vi "Main.vi"(11 "Module Admin":refnum<class "Delacor_lib_QMH_Module Admin.lvclass">) -> ()   [LabVIEW 2022 SP3, in "MainPanel.lvlib"]
doc: "This template is based off of the Queued Message Handler design pattern and the Queued Message Handler project template that ships with LabVIEW.\n\nThe main difference is that the queue is private to this module and communication between modules is performed via Broadcast and Request events.\n\nRequest events are wrapped in public API methods and are handled in the Event Handling Loop (EHL) of this VI. Any module can register for Broadcast events sent by this module. The EHL generates messages based on user interface actions.\n\nThe Message Handling Loop (MHL) processes messages generated by the EHL, or by other messages. The messages are string values, so new messages can be added easily to the Message Cases case structure in the MHL. Each message cluster can also provide an optional value for Message Data, which is a variant that can be converted to whatever message-specific data is required.\n_____\nBased on DQMH Project Template 7.0.1.1316."
uses:
  MainPanel.lvlib
  <vilib>/Delacor/Delacor QMH/Libraries/Module Admin_class/Delacor_lib_QMH_Module Admin.lvclass
  Module Data--cluster.ctl
  Do Something Argument--cluster.ctl
  <vilib>/Delacor/Delacor QMH/Libraries/Message Queue_class/Delacor_lib_QMH_Message Queue.lvclass/Delacor_lib_QMH_Message Queue.ctl
  Do Something Else Argument--cluster.ctl
  Do Something Else and Wait for Reply Argument--cluster.ctl
  Do Something Else and Wait (Reply Payload)--cluster.ctl
  Stop Argument--cluster.ctl
  <vilib>/Delacor/Delacor QMH/Libraries/Module Admin_class/Delacor_lib_QMH_Module Admin.lvclass/Delacor_lib_QMH_Module Admin.ctl
  Prepare Argument--cluster.ctl
  Configure Argument--cluster.ctl
  Request UI Display Argument--cluster.ctl
  Framework/UI Manager/Module Display Scenarios.ctl
  Request UI Display (Reply Payload)--cluster.ctl
  Update UI Argument--cluster.ctl
  <vilib>/Utility/miscctls.llb/LVPointTypeDef.ctl
  <vilib>/Delacor/Delacor QMH/Libraries/Message Queue_class/Delacor_lib_QMH_Enqueue Message (Single).vi
  <vilib>/Delacor/Delacor QMH/Libraries/Module Admin_class/Delacor_lib_QMH_Get External Launch.vi
  <vilib>/Delacor/Delacor QMH/Libraries/Message Queue_class/Delacor_lib_QMH_Message Queue.lvclass
  Libraries/hse-libraries/Source/hse-configuration/config-ini/config-ini.lvclass
  Framework/UI Manager/UI Manager.lvlib
  <vilib>/Hampel Software Engineering/HSE Logger/hse-logger.lvlib
  Libraries/hse-libraries/Source/hse-dqmh/hse-dqmh.lvlib
panel:
  in  "Run Model":bool
  out "error out":errorcluster
  out "X":dbl
  out "Status":string
  in  "Simulate MHL Error":bool
  in  "Simulate EHL Error":bool
  in  "Do Something Else <Replace Me>":bool
  in  "Do Something <Replace Me>":bool
  # "These controls have associated \"Value Changed\" events configured in the Event Structure on the diagram.\n\nReplace them (and reconfigure the Event Structure) with the controls you need for your application. \n\nOther processes communicate with this Module via its Public API (wrappers for its Request Events).\n\nThis Module communicates with other processes via its Broadcast Events.\nAny process that wants to receive these messages can register for this module's Broadcast events."
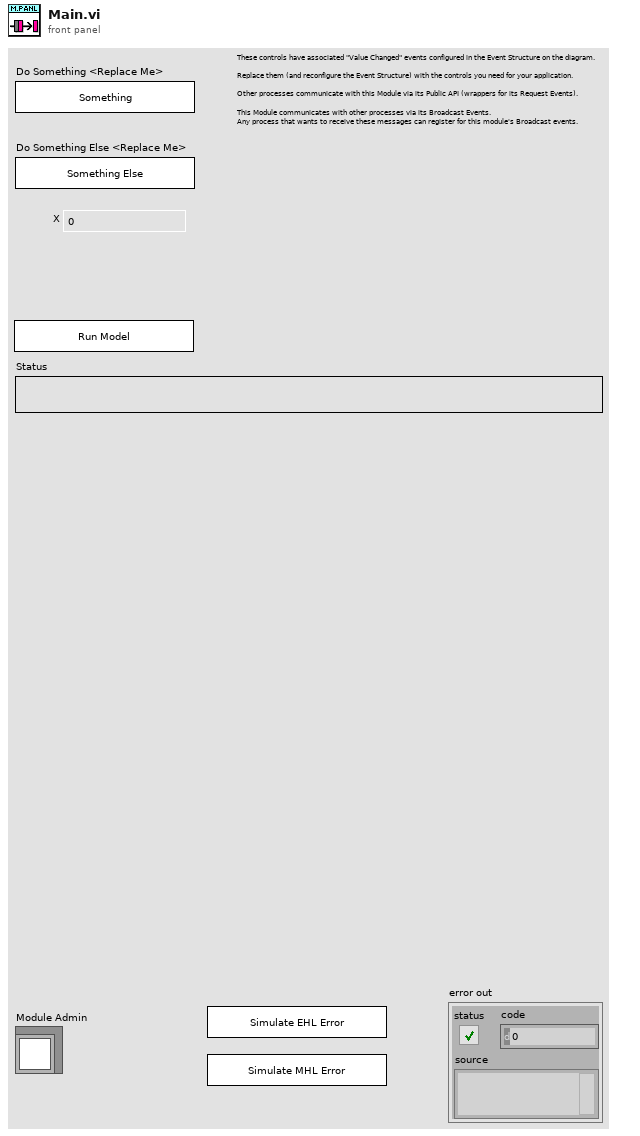
[diagram p1: front panel]
types:
  T1 = typedef "MainPanel.lvlib/Request Events--cluster.ctl" = cluster{"Stop Module":refnum<user-event>, "Do Something":refnum<user-event>, "Do Something Else":refnum<user-event>, "Do Something Else and Wait for Reply":refnum<user-event>, "Show Panel":refnum<user-event>, "Hide Panel":refnum<user-event>, "Get Module Execution Status":refnum<user-event>, "Show Diagram":refnum<user-event>, "Prepare":refnum<user-event>, "Configure":refnum<user-event>, "Request UI Display":refnum<user-event>, "Private":cluster{"Update UI":refnum<user-event>}}
  T2 = typedef "MainPanel.lvlib/Module Data--cluster.ctl" = cluster{"Status":string, "Py Session":refnum<k35>, "Py Script Path":path}
  T3 = typedef "MainPanel.lvlib/Do Something Argument--cluster.ctl" = cluster{"Do Something Msg":string}
  T4 = typedef "MainPanel.lvlib/Do Something Else Argument--cluster.ctl" = cluster{"Do Something Else Msg":string, "X":dbl}
  T5 = typedef "MainPanel.lvlib/Do Something Else and Wait for Reply Argument--cluster.ctl" = cluster{"Do Something Else Msg":string, "X":dbl, "Wait Notifier":refnum<notifier>, "wait for reply":bool}
  T6 = enum32{"invalid lock state", "Not Locked", "Locked (No Password)", "Password-protected"}
  T7 = typedef "MainPanel.lvlib/Stop Argument--cluster.ctl" = cluster{"Origin":string, "Exit via Stop Module Req?":bool, "Wait for Module to stop?":bool}
  T8 = typedef "MainPanel.lvlib/Prepare Argument--cluster.ctl" = cluster{"Boolean":bool}
  T9 = typedef "MainPanel.lvlib/Configure Argument--cluster.ctl" = cluster{"Boolean":bool}
  T10 = typedef "MainPanel.lvlib/Request UI Display Argument--cluster.ctl" = cluster{"Scenario":T11, "Wait Notifier":refnum<notifier>, "wait for reply":bool}
  T11 = typedef "UI Manager.lvlib/Module Display Scenarios.ctl" = enum16{"Stand-Alone", "Managed"}
  T12 = typedef "MainPanel.lvlib/Update UI Argument--cluster.ctl" = cluster{"Update":bool}
  T13 = typedef "LVPointTypeDef.ctl" = cluster{"Horizontal":i16, "Vertical":i16}
  T14 = enum32{"Invalid", "Standard", "Closed", "Hidden", "Minimized", "Maximized"}
  T15 = typedef "MainPanel.lvlib/Do Something Else and Wait (Reply Payload)--cluster.ctl" = cluster{"Value":dbl, "error":errorcluster}
  T16 = typedef "MainPanel.lvlib/Request UI Display (Reply Payload)--cluster.ctl" = cluster{"Accept":bool, "error":errorcluster}
  T17 = typedef "hse-dqmh.lvlib/System Message Source.ctl" = enum16{"module", "application", "network"}
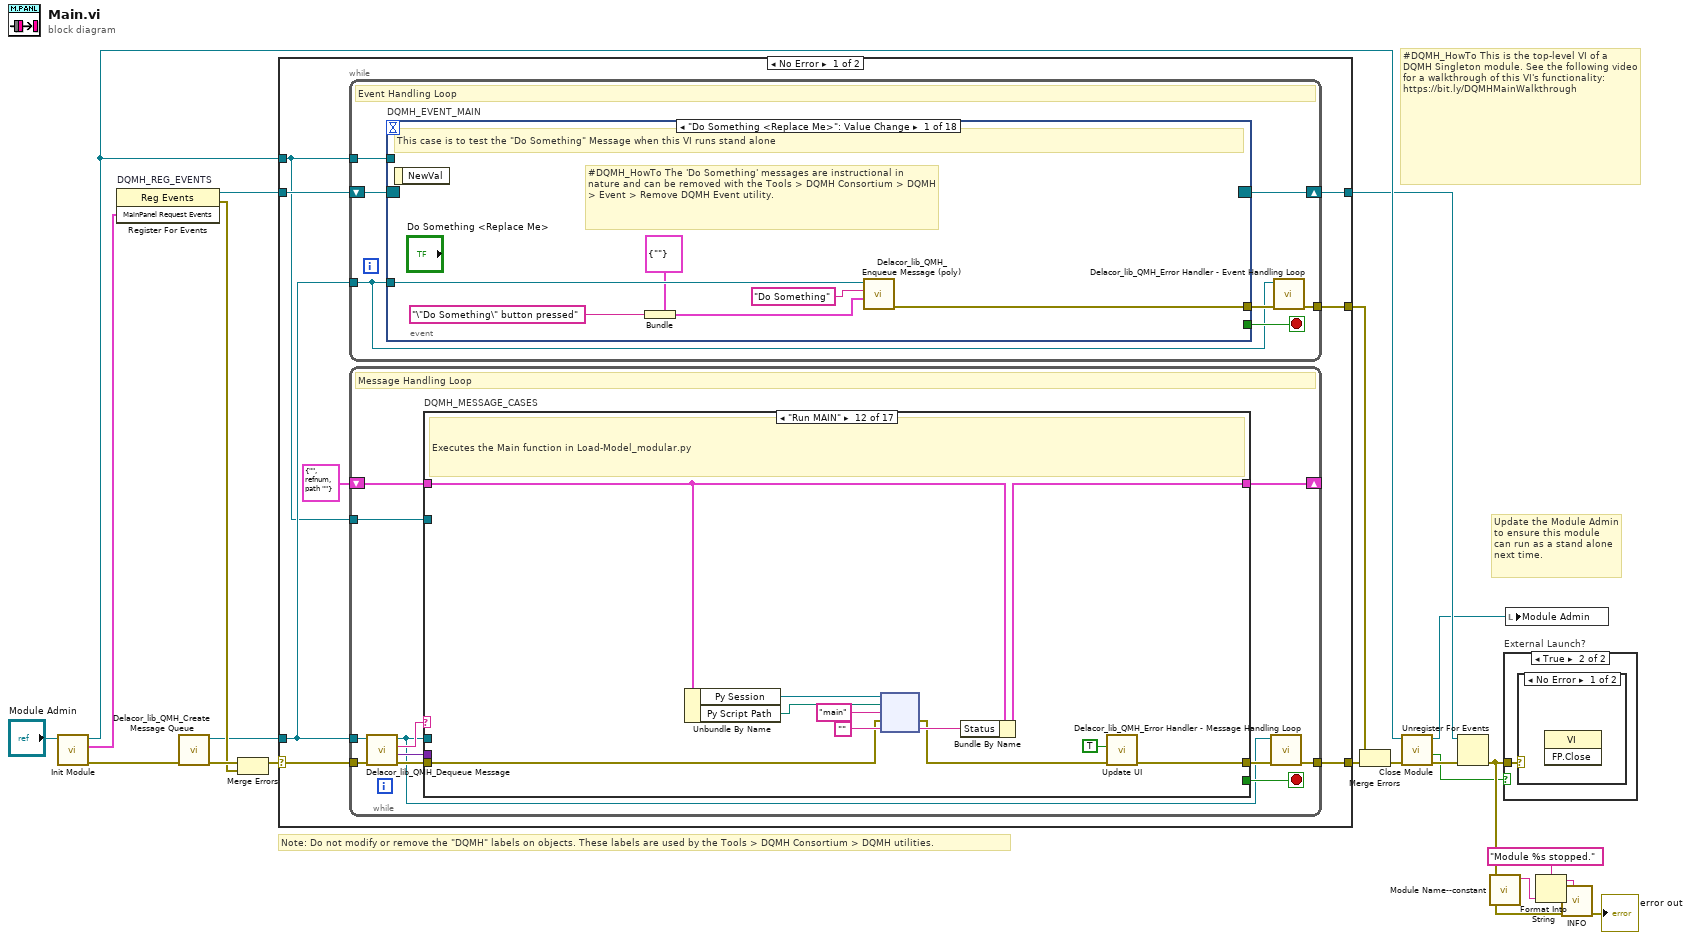
[diagram p0: block diagram]
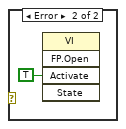
[diagram p3: hidden frame]
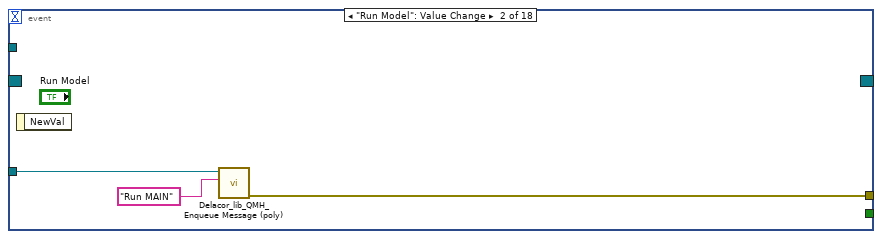
[diagram p4: hidden frame]
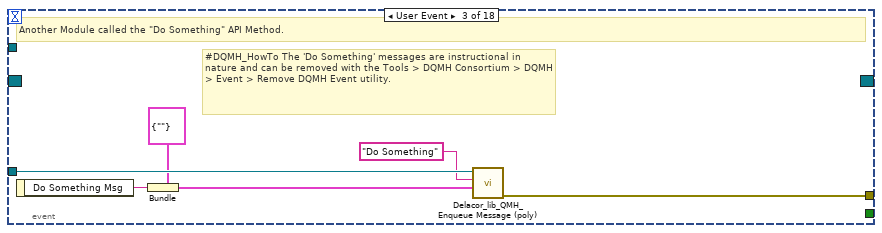
[diagram p5: hidden frame]
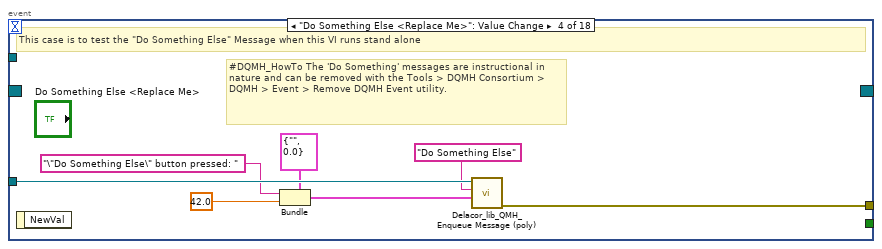
[diagram p6: hidden frame]
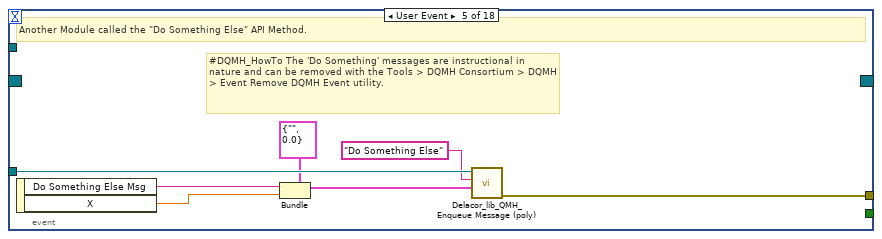
[diagram p7: hidden frame]
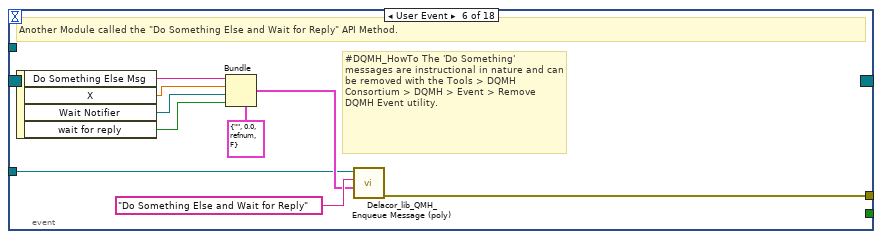
[diagram p8: hidden frame]
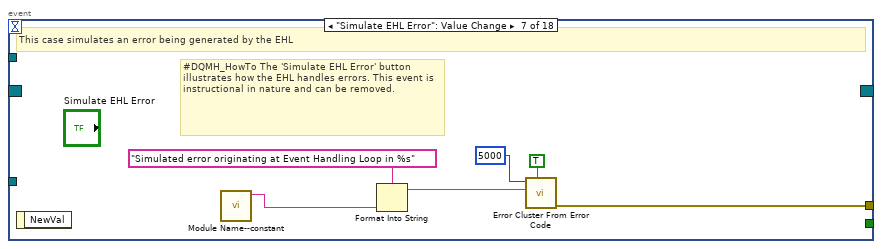
[diagram p9: hidden frame]
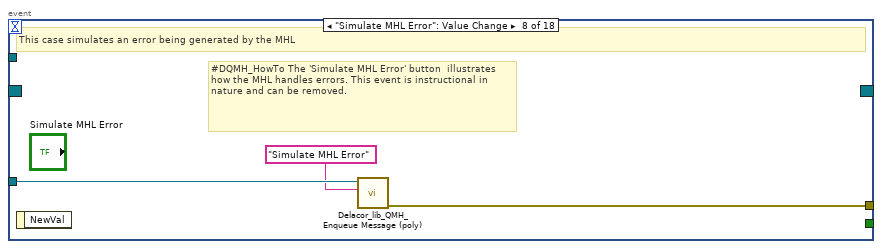
[diagram p10: hidden frame]
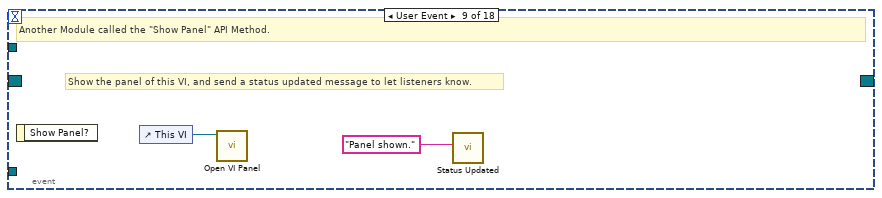
[diagram p11: hidden frame]
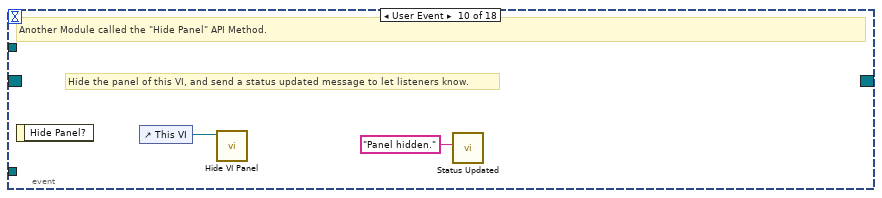
[diagram p12: hidden frame]
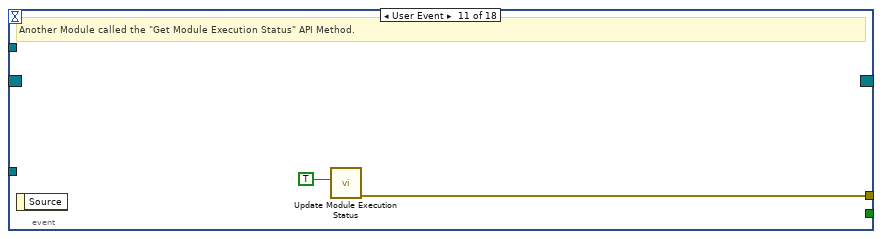
[diagram p13: hidden frame]
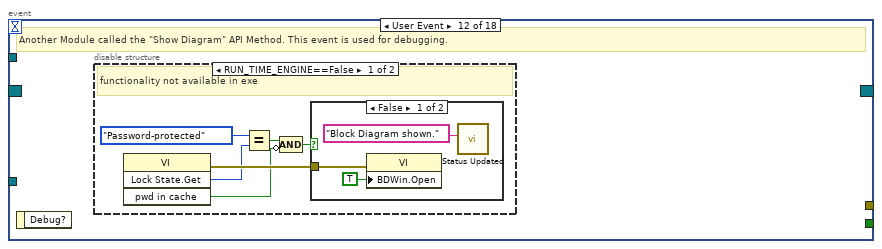
[diagram p14: hidden frame]
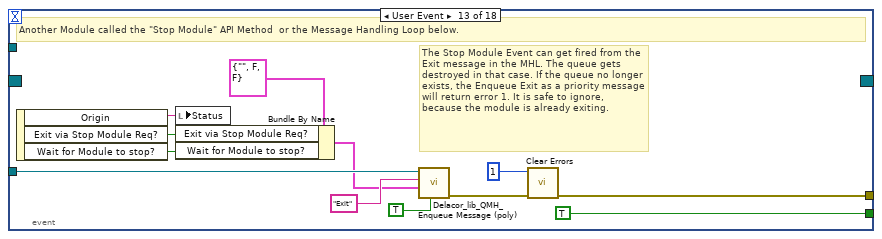
[diagram p17: hidden frame]
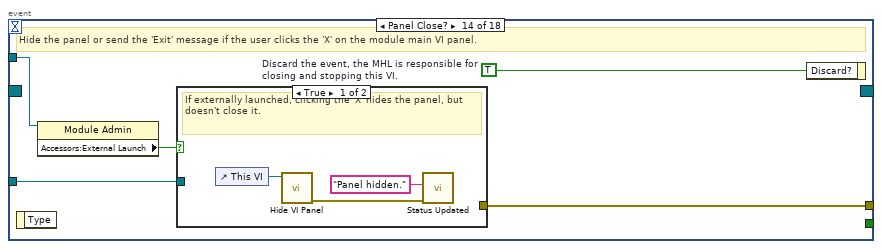
[diagram p18: hidden frame]
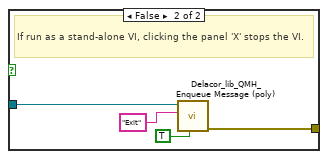
[diagram p19: hidden frame]
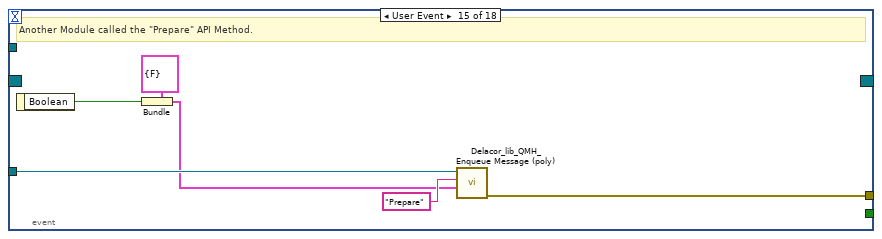
[diagram p20: hidden frame]
diagram:
  # "#DQMH_HowTo This is the top-level VI of a DQMH Singleton module. See the following video for a walkthrough of this VI's functionality: https://bit.ly/DQMHMainWalkthrough"
  # "Note: Do not modify or remove the \"DQMH\" labels on objects. These labels are used by the Tools > DQMH Consortium > DQMH utilities."
  # "Update the Module Admin to ensure this module can run as a stand alone next time."
  n1 = call "Init Module.vi"("Singleton Module Admin in"="Module Admin") -> ("error out"=w20:errorcluster, "MainPanel Request Events"=w9:T1, "Singleton Module Admin out"=w12:refnum<class "Delacor_lib_QMH_Module Admin.lvclass">)  [unwired: 8 in]
  n2 = register-events "DQMH_REG_EVENTS"(w9) -> (reference out=w10:refnum<event-registration>, error out=w13:errorcluster)  [unwired: 2 in]
  n3 = call <vilib>:"Delacor_lib_QMH_Create Message Queue.vi"("error in"=w20) -> ("error out"=w15:errorcluster, "Message Queue"=w8:refnum<class "Delacor_lib_QMH_Message Queue.lvclass">)  [unwired: 9 in]
  n4 = Merge Errors(w15, w13) -> (w14:errorcluster)
  n5 = case shown="No Error" w14 {
    selector: w14 -> [w27 w372]
    tunnel: [w29 w371] -> w21
    tunnel: [w26 w370] -> w11
    tunnel: w10 -> [w24 w370]
    tunnel: w8 -> [w23 w365]
    tunnel: [w28 _] -> w18
    tunnel: w12 -> [w22 w366]
    frame No Error {
      n6 = while {
        tunnel: w23 -> [w30]
        shift-right: [w33] -> w26
        shift-left: w24 -> [w34]
        tunnel: [w35] -> w28
        tunnel: w22 -> [w31]
        stop <- w32 stop-if-true
        # "Event Handling Loop"
        n7 = event "DQMH_EVENT_MAIN" shown="[0] \"Do Something <Replace Me>\": Value Change" {
          selector: w34 -> [_ _ _ _ _ _ _ _ _ _ _ _ _ _ _ _ _ _]
          dyn-events: [_ _ _ _ _ _ _ _ _ _ _ _ _ _ _ _ _ _] -> w33
          timeout: _ -> [_ _ _ _ _ _ _ _ _ _ _ _ _ _ _ _ _ _]
          tunnel: [_ _ _ _ _ _ _ _ _ _ _ _ TRUE ("Discard?") _ _ _ _ _] -> w32
          tunnel: w30 -> [w41 w44 w50 w57 w64 w67 _ w82 _ _ _ _ w106 w113 w128 w134 w142 w148]
          tunnel: [w42 w43 w51 w58 w65 w74 w80 w83 _ _ w89 _ w109 w115 w123 w129 w135 w143] -> w36
          tunnel: w31 -> [_ _ _ _ _ _ _ _ _ _ _ _ _ w112 _ _ _ _]
          event "Do Something <Replace Me>": Value Change {
            # "#DQMH_HowTo The 'Do Something' messages are instructional in nature and can be removed with the Tools > DQMH Consortium > DQMH > Event > Remove DQMH Event utility."
            # "This case is to test the \"Do Something\" Message when this VI runs stand alone"
            n8 = event-data() -> ()  [unwired: 1 in, 1 out]
            n9 = Bundle(cluster=T3 {"Do Something Msg"=""} ("Do Something Argument"), "Do Something Msg"="\"Do Something\" button pressed" ("\"Do Something\" button pressed")) -> (w37:T3)
            n10 = call-poly <vilib>:"Delacor_lib_QMH_Enqueue Message (poly).vi"("Message Data"=w37, "Message"="Do Something", "Message Queue in"=w41) -> ("error out"=w42:errorcluster)  [unwired: 7 in, 1 out]
          }
          event "Run Model": Value Change {
            n11 = event-data() -> ()  [unwired: 1 in, 1 out]
            n12 = call-poly <vilib>:"Delacor_lib_QMH_Enqueue Message (poly).vi"("Message"="Run MAIN", "Message Queue in"=w44) -> ("error out"=w43:errorcluster)  [unwired: 8 in, 1 out]
          }
          event User Event {
            # "#DQMH_HowTo The 'Do Something' messages are instructional in nature and can be removed with the Tools > DQMH Consortium > DQMH > Event > Remove DQMH Event utility."
            # "Another Module called the \"Do Something\" API Method."
            n13 = event-data() -> ("Do Something Msg"=w47:string)  [unwired: 1 in]
            n14 = Bundle(cluster=T3 {"Do Something Msg"=""} ("Do Something Argument"), "Do Something Msg"=w47) -> (w46:T3)
            n15 = call-poly <vilib>:"Delacor_lib_QMH_Enqueue Message (poly).vi"("Message Data"=w46, "Message"="Do Something", "Message Queue in"=w50) -> ("error out"=w51:errorcluster)  [unwired: 7 in, 1 out]
          }
          event "Do Something Else <Replace Me>": Value Change {
            # "#DQMH_HowTo The 'Do Something' messages are instructional in nature and can be removed with the Tools > DQMH Consortium > DQMH > Event > Remove DQMH Event utility."
            # "This case is to test the \"Do Something Else\" Message when this VI runs stand alone"
            n16 = event-data() -> ()  [unwired: 1 in, 1 out]
            n17 = Bundle(cluster=T4 {"Do Something Else Msg"="", "X"=0.0} ("Do Something Else Argument"), "Do Something Else Msg"="\"Do Something Else\" button pressed: " ("\"Do Something Else\" button pressed"), "X"=42.0) -> (w54:T4)
            n18 = call-poly <vilib>:"Delacor_lib_QMH_Enqueue Message (poly).vi"("Message Data"=w54, "Message"="Do Something Else", "Message Queue in"=w57) -> ("error out"=w58:errorcluster)  [unwired: 7 in, 1 out]
          }
          event User Event {
            # "#DQMH_HowTo The 'Do Something' messages are instructional in nature and can be removed with the Tools > DQMH Consortium > DQMH > Event Remove DQMH Event utility."
            # "Another Module called the \"Do Something Else\" API Method."
            n19 = event-data() -> ("Do Something Else Msg"=w60:string, "X"=w59:dbl)  [unwired: 1 in]
            n20 = Bundle(cluster=T4 {"Do Something Else Msg"="", "X"=0.0} ("Do Something Else Argument"), "Do Something Else Msg"=w60, "X"=w59) -> (w61:T4)
            n21 = call-poly <vilib>:"Delacor_lib_QMH_Enqueue Message (poly).vi"("Message Data"=w61, "Message"="Do Something Else", "Message Queue in"=w64) -> ("error out"=w65:errorcluster)  [unwired: 7 in, 1 out]
          }
          event User Event {
            # "#DQMH_HowTo The 'Do Something' messages are instructional in nature and can be removed with the Tools > DQMH Consortium > DQMH > Event > Remove DQMH Event utility."
            # "Another Module called the \"Do Something Else and Wait for Reply\" API Method."
            n22 = event-data() -> ("Do Something Else Msg"=w70:string, "X"=w69:dbl, "Wait Notifier"=w68:refnum<notifier>, "wait for reply"=w66:bool)  [unwired: 1 in]
            n23 = Bundle(cluster=T5 {"Do Something Else Msg"="", "X"=0.0, "Wait Notifier"=refnum, "wait for reply"=FALSE} ("Do Something Else and Wait for Reply Argument"), "Do Something Else Msg"=w70, "X"=w69, "Wait Notifier"=w68, "wait for reply"=w66) -> (w71:T5)
            n24 = call-poly <vilib>:"Delacor_lib_QMH_Enqueue Message (poly).vi"("Message Data"=w71, "Message"="Do Something Else and Wait for Reply", "Message Queue in"=w67) -> ("error out"=w74:errorcluster)  [unwired: 7 in, 1 out]
          }
          event "Simulate EHL Error": Value Change {
            # "#DQMH_HowTo The 'Simulate EHL Error' button  illustrates how the EHL handles errors. This event is instructional in nature and can be removed."
            # "This case simulates an error being generated by the EHL"
            n25 = event-data() -> ()  [unwired: 1 in, 1 out]
            n26 = call "Module Name--constant.vi"() -> ("Module Name"=w77:string)  [unwired: 11 in]
            n27 = Format Into String(format string="Simulated error originating at Event Handling Loop in %s", w77) -> (resulting string=w78:string)  [unwired: 2 in, 1 out]
            n28 = call <vilib>:"Error Cluster From Error Code.vi"("show call chain? (False)"=TRUE, "error message (\"\")"=w78, "error code (0)"=5000) -> ("error out"=w80:errorcluster)  [unwired: 6 in]
          }
          event "Simulate MHL Error": Value Change {
            # "#DQMH_HowTo The 'Simulate MHL Error' button  illustrates how the MHL handles errors. This event is instructional in nature and can be removed."
            # "This case simulates an error being generated by the MHL"
            n29 = event-data() -> ()  [unwired: 1 in, 1 out]
            n30 = call-poly <vilib>:"Delacor_lib_QMH_Enqueue Message (poly).vi"("Message"="Simulate MHL Error", "Message Queue in"=w82) -> ("error out"=w83:errorcluster)  [unwired: 8 in, 1 out]
          }
          event User Event {
            # "Show the panel of this VI, and send a status updated message to let listeners know."
            # "Another Module called the \"Show Panel\" API Method."
            n31 = event-data() -> ()  [unwired: 1 in, 1 out]
            n32 = control-ref of="This VI"() -> (w85:refnum<vi>)
            n33 = call "Open VI Panel.vi"("VI"=w85) -> ()  [unwired: 10 in, 1 out]
            n34 = call "Status Updated.vi"("Status"="Panel shown." ("format string")) -> ()  [unwired: 10 in, 1 out]
          }
          event User Event {
            # "Hide the panel of this VI, and send a status updated message to let listeners know."
            # "Another Module called the \"Hide Panel\" API Method."
            n35 = event-data() -> ()  [unwired: 1 in, 1 out]
            n36 = control-ref of="This VI"() -> (w87:refnum<vi>)
            n37 = call "Hide VI Panel.vi"("VI"=w87) -> ()  [unwired: 10 in, 1 out]
            n38 = call "Status Updated.vi"("Status"="Panel hidden." ("format string")) -> ()  [unwired: 10 in, 1 out]
          }
          event User Event {
            # "Another Module called the \"Get Module Execution Status\" API Method."
            n39 = event-data() -> ()  [unwired: 1 in, 1 out]
            n40 = call "Update Module Execution Status.vi"("Running?"=TRUE) -> ("error out"=w89:errorcluster)  [unwired: 10 in]
          }
          event User Event {
            # "Another Module called the \"Show Diagram\" API Method. This event is used for debugging."
            n41 = event-data() -> ()  [unwired: 1 in, 1 out]
            n42 = disable-structure shown="RUN_TIME_ENGINE==False" {
              frame condition #0 (active) {
                # "functionality not available in exe"
                n43 = invoke on="Invoke Node" class="VI" method="Lock State.Get"() -> (error out=w95:errorcluster, "Get Lock State"=w94:T6, "pwd in cache"=w91:bool)  [unwired: 4 in, 1 out]
                n44 = Equal?(x=T6."Password-protected", y=w94) -> (x = y?=w92:bool)
                n45 = Compound Arithmetic op=AND(w92, invert w91) -> (w90:bool)
                n46 = case shown="False" w90 {
                  tunnel: w95 -> [w98 _]
                  frame False {
                    n47 = property on="Property Node" class="VI"(error in=w98, "BDWin.Open"=TRUE ("Block Diagram Window:Open")) -> ()  [unwired: 1 in, 2 out]
                    n48 = call "Status Updated.vi"("Status"="Block Diagram shown." ("format string")) -> ()  [unwired: 10 in, 1 out]
                  }
                  frame True {
                    # "Password-protected VI, and the password is not in the cache. Do not show the diagram."
                  }
                }
              }
              frame condition #1 {
              }
            }
          }
          event User Event {
            # "The Stop Module Event can get fired from the Exit message in the MHL. The queue gets destroyed in that case. If the queue no longer exists, the Enqueue Exit as a priority message will return error 1. It is safe to ignore, because the module is already exiting."
            # "Another Module called the \"Stop Module\" API Method  or the Message Handling Loop below."
            n49 = event-data() -> ("Origin"=w105:string, "Exit via Stop Module Req?"=w101:bool, "Wait for Module to stop?"=w100:bool)  [unwired: 1 in]
            n50 = local write "Status"(w105) -> ()
            n51 = Bundle By Name(cluster=T7 {"Origin"="", "Exit via Stop Module Req?"=FALSE, "Wait for Module to stop?"=FALSE} ("Stop Argument"), "Exit via Stop Module Req?"=w101, "Wait for Module to stop?"=w100) -> (w99:T7)
            n52 = call-poly <vilib>:"Delacor_lib_QMH_Enqueue Message (poly).vi"("Priority Message? (F)"=TRUE, "Message Data"=w99, "Message"="Exit", "Message Queue in"=w106) -> ("error out"=w110:errorcluster)  [unwired: 6 in, 1 out]
            n53 = call <vilib>:"Clear Errors.vi"("error in (no error)"=w110, "specific error code to clear (0: all)"=1) -> ("error out"=w109:errorcluster)  [unwired: 4 in, 1 out]
          }
          event Panel Close? {
            w114 = TRUE  # Discard the event, the MHL is responsible for closing and stopping this VI.
            # "Hide the panel or send the 'Exit' message if the user clicks the 'X' on the module main VI panel."
            n54 = event-data() -> ()  [unwired: 1 in, 1 out]
            n55 = property on="Property Node" class="Module Admin"(reference=w112) -> ("Accessors:External Launch"=w111:bool)  [unwired: 1 in, 2 out]
            n56 = case shown="True" w111 {
              tunnel: w113 -> [_ w121]
              tunnel: [_ w122] -> w115
              frame True {
                # "If externally launched, clicking the 'X' hides the panel, but doesn't close it."
                n57 = control-ref of="This VI"() -> (w118:refnum<vi>)
                n58 = call "Hide VI Panel.vi"("VI"=w118) -> ("error out"=w116:errorcluster)  [unwired: 10 in]
                n59 = call "Status Updated.vi"("error in"=w116, "Status"="Panel hidden." ("format string")) -> ()  [unwired: 9 in, 1 out]
              }
              frame False {
                # "If run as a stand-alone VI, clicking the panel 'X' stops the VI."
                n60 = call-poly <vilib>:"Delacor_lib_QMH_Enqueue Message (poly).vi"("Priority Message? (F)"=TRUE, "Message"="Exit", "Message Queue in"=w121) -> ("error out"=w122:errorcluster)  [unwired: 7 in, 1 out]
              }
            }
            n61 = event-data ("Event Filter Node")("Discard?"=w114) -> ()  [unwired: 1 in, 1 out]
          }
          event User Event {
            # "Another Module called the \"Prepare\" API Method."
            n62 = event-data() -> ("Boolean"=w124:bool)  [unwired: 1 in]
            n63 = Bundle(cluster=T8 {"Boolean"=FALSE} ("Prepare Argument"), "Boolean"=w124) -> (w125:T8)
            n64 = call-poly <vilib>:"Delacor_lib_QMH_Enqueue Message (poly).vi"("Message Data"=w125, "Message"="Prepare", "Message Queue in"=w128) -> ("error out"=w123:errorcluster)  [unwired: 7 in, 1 out]
          }
          event User Event {
            # "Another Module called the \"Configure\" API Method."
            n65 = event-data() -> ("Boolean"=w130:bool)  [unwired: 1 in]
            n66 = Bundle(cluster=T9 {"Boolean"=FALSE} ("Configure Argument"), "Boolean"=w130) -> (w131:T9)
            n67 = call-poly <vilib>:"Delacor_lib_QMH_Enqueue Message (poly).vi"("Message Data"=w131, "Message"="Configure", "Message Queue in"=w134) -> ("error out"=w129:errorcluster)  [unwired: 7 in, 1 out]
          }
          event User Event {
            # "Another Module called the \"Request UI Display\" API Method."
            n68 = event-data() -> ("Scenario"=w138:T11, "Wait Notifier"=w137:refnum<notifier>, "wait for reply"=w136:bool)  [unwired: 1 in]
            n69 = Bundle(cluster=T10 {"Scenario"=enum."Stand-Alone", "Wait Notifier"=refnum, "wait for reply"=FALSE} ("Request UI Display Argument"), "Scenario"=w138, "Wait Notifier"=w137, "wait for reply"=w136) -> (w139:T10)
            n70 = call-poly <vilib>:"Delacor_lib_QMH_Enqueue Message (poly).vi"("Message Data"=w139, "Message"="Request UI Display", "Message Queue in"=w142) -> ("error out"=w135:errorcluster)  [unwired: 7 in, 1 out]
          }
          event User Event {
            # "This module called the \"Private.Update UI\" private request."
            n71 = event-data() -> ("Update"=w144:bool)  [unwired: 1 in]
            n72 = Bundle(cluster=T12 {"Update"=FALSE} ("Update UI Argument"), "Update"=w144) -> (w145:T12)
            n73 = call-poly <vilib>:"Delacor_lib_QMH_Enqueue Message (poly).vi"("Message Data"=w145, "Message"="Update UI", "Message Queue in"=w148) -> ("error out"=w143:errorcluster)  [unwired: 7 in, 1 out]
          }
        }
        n74 = call-dynamic "Delacor_lib_QMH_Error Handler - Event Handling Loop.vi"("error in"=w36, "Message Queue in"=w30) -> ("dup error in"=w35:errorcluster)  [unwired: 8 in, 1 out]
      }
      n75 = while {
        tunnel: w23 -> [w149]
        shift-right: [w157] -> _
        shift-left: T2 {"Status"="", "Py Session"=refnum, "Py Script Path"=path ""} ("Data Cluster") -> [w158]
        tunnel: w27 -> [w160]
        tunnel: [w152] -> w29
        tunnel: w22 -> [w153]
        stop <- w156 stop-if-true
        # "Message Handling Loop"
        n76 = call-dynamic "Delacor_lib_QMH_Dequeue Message.vi"("error in"=w160, "Message Queue in"=w149) -> ("error out"=w159:errorcluster, "Message Data"=w154:variant, "Message"=w155:string, "Message Queue out"=w150:refnum<class "Delacor_lib_QMH_Message Queue.lvclass">)  [unwired: 6 in]
        n77 = case "DQMH_MESSAGE_CASES" shown="\"Run MAIN\"" w155 {
          selector: w155 -> [_ _ _ _ _ _ _ _ _ _ _ _ _ _ _ _ w360]
          tunnel: w150 -> [_ _ _ _ _ _ _ _ _ _ _ _ _ _ w324 w350 _]
          tunnel: w159 -> [w183 w187 w195 w204 w223 w243 w246 w273 w290 w293 w296 w300 w309 w318 w331 w354 w363]
          tunnel: [w162 w187 w193 w203 w222 w235 w244 w268 w289 w292 w295 w298 w309 w317 w327 w351 w364] -> w151
          tunnel: w158 -> [w172 w186 w192 w202 w219 w242 w260 w272 w286 w291 w294 w307 w308 w315 w326 w339 w361]
          tunnel: [w171 w186 w192 w202 w219 w237 w260 w272 w286 w291 w294 w302 w308 w315 w326 w339 w361] -> w157
          tunnel: [_ _ _ _ _ _ _ _ _ _ _ _ _ _ _ w349 _] -> w156
          tunnel: w154 -> [_ _ w191 w199 w216 w241 _ w270 w288 _ _ _ _ _ w325 w348 _]
          tunnel: w153 -> [w173 _ _ _ _ _ _ _ _ _ _ _ _ _ w323 w343 _]
          frame "Initialize" {
            # "#CodeNeeded - Initialize the appearance of the front panel."
            # "#CodeNeeded - Initialize your state data here."
            # "Initialize - Any operation that needs to be done before the module can receive messages. Synchronize Caller Events.vi will inform Start Module.vi that the module has launched and is ready to receive messages. Module Did Init.vi will broadcast that the module initialized."
            n78 = call "Synchronize Caller Events.vi"("error in"=w183, "Singleton Module Admin in"=w173) -> ("error out"=w182:errorcluster, "Singleton Module Admin out"=w168:refnum<class "Delacor_lib_QMH_Module Admin.lvclass">)  [unwired: 8 in]
            n79 = property on="Property Node" class="Module Admin"(reference=w168) -> ("Accessors:External Launch"=w177:bool)  [unwired: 1 in, 2 out]
            n80 = Select(t=T14."Hidden" ("State"), s=w177, f=T14."Standard" ("State")) -> (s? t:f=w174:T14)
            n81 = call "Module Name--constant.vi"() -> ("Module Name"=w169:string)  [unwired: 11 in]
            n82 = call "Module Name--constant.vi"() -> ("Module Name"=w180:string)  [unwired: 11 in]
            n83 = property on="Property Node" class="VI"("Front Panel.Title"=w180) -> (reference out=w179:refnum<vi>, error out=w185:errorcluster)  [unwired: 2 in]
            n84 = call "Module Did Init.vi"("error in"=w182, "Initialized?"=TRUE, "Origin"=w169) -> ("error out"=w181:errorcluster)  [unwired: 8 in]
            n85 = invoke on="Invoke Node" class="VI" method="FP.Open"(reference=w179, error in=w185, "State"=w174) -> (reference out=w178:refnum<vi>, error out=w184:errorcluster)  [unwired: 2 in, 3 out]
            n86 = Bundle By Name(cluster=w172, "Status"="Initial Message" ("Initial Message")) -> (w171:T2)
            n87 = invoke on="Invoke Node" class="VI" method="FP.Center"(reference=w178, error in=w184) -> ()  [unwired: 1 in, 3 out]
            n88 = property on="Pane" class="Pane"("Origin"=T13 {"Horizontal"=0, "Vertical"=0}) -> ()  [unwired: 2 in, 2 out]
            n89 = Format Into String(format string="Module %s started.", w169) -> (resulting string=w165:string)  [unwired: 2 in, 1 out]
            n90 = call <vilib>:"INFO.vi"("Message"=w165, "error in"=w181) -> ("error out"=w163:errorcluster)  [unwired: 9 in]
            n91 = call "Update UI.vi"("error in"=w163, "Update"=TRUE) -> ("error out"=w162:errorcluster)  [unwired: 9 in]
          }
          frame "---Module Specific---" {
            # "Separator -- The following cases handle messages specific to this Module."
          }
          frame "Do Something" {
            # "#DQMH_HowTo The 'Do Something' messages are instructional in nature and can be removed with the Tools > DQMH Consortium > DQMH > Event > Remove DQMH Event utility."
            # "Do Something - Replace this message with functionality for your own application. Note that this message also fires the \"Did Something\" broadcast event."
            n92 = Variant To Data(error in=w195, type=T3 {"Do Something Msg"=""} ("Do Something Argument"), Variant=w191) -> (data=w190:T3, error out=w194:errorcluster)
            n93 = Unbundle By Name(w190) -> ("Do Something Msg"=w188:string)
            n94 = call "Did Something.vi"("error in"=w194, "Did Something Msg"=w188) -> ("error out"=w193:errorcluster)  [unwired: 9 in]
            n95 = local write "Status"(w188) -> ()
            n96 = call "Status Updated.vi"("Status"=w188) -> ()  [unwired: 10 in, 1 out]
          }
          frame "Do Something Else" {
            # "#DQMH_HowTo The 'Do Something' messages are instructional in nature and can be removed with the Tools > DQMH Consortium > DQMH > Event > Remove DQMH Event utility."
            # "Do Something Else - Replace this message with functionality for your own application."
            n97 = Variant To Data(error in=w204, type=T4 {"Do Something Else Msg"="", "X"=0.0} ("Do Something Else Argument"), Variant=w199) -> (data=w200:T4, error out=w203:errorcluster)
            n98 = Unbundle By Name(w200) -> ("Do Something Else Msg"=w198:string, "X"=w197:dbl)
            "X" <- w197
            n99 = Format Into String(initial string=w198, w197) -> (resulting string=w196:string)  [unwired: 2 in, 1 out]
            n100 = local write "Status"(w196) -> ()
            n101 = call "Status Updated.vi"("Status"=w196) -> ()  [unwired: 10 in, 1 out]
          }
          frame "Do Something Else and Wait for Reply" {
            w211 = "X(%.2f)+Offset(%.2f)=%.2f"  # status message format string
            # "#DQMH_HowTo The 'Do Something' messages are instructional in nature and can be removed."
            # "Send back X with a random offset"
            # "Do Something Else and Wait for Reply - Replace this message with functionality for your own application. Note that this message must fire a notifier to let callers know it has finished execution, and it returns an error if the 'Value' is negative."
            n102 = Variant To Data(error in=w223, type=T5 {"Do Something Else Msg"="", "X"=0.0, "Wait Notifier"=refnum, "wait for reply"=FALSE} ("Do Something Else and Wait for Reply Argument"), Variant=w216) -> (data=w217:T5, error out=w221:errorcluster)
            n103 = Unbundle By Name(w217) -> ("Wait Notifier"=w205:refnum<notifier>, "Do Something Else Msg"=w215:string, "X"=w212:dbl, "wait for reply"=w208:bool)
            n104 = Random Number (0-1)() -> (number: 0 to 1=w213:dbl)
            n105 = Add(x=w213, y=w212) -> (x+y=w207:dbl)
            n106 = Less Than 0?(x=w207) -> (x < 0?=w210:bool)
            n107 = local write "X"(w212) -> ()
            n108 = case shown="True" w210 {
              tunnel: [_ w233] -> w220
              frame False {
              }
              frame True {
                n109 = call <vilib>:"Error Cluster From Error Code.vi"("show call chain? (False)"=TRUE, "error message (\"\")"="The 'Something Else and Wait for Reply' message generated a negative number, which is considered an error condition.", "error code (0)"=5000) -> ("error out"=w233:errorcluster)  [unwired: 6 in]
              }
            }
            n110 = Format Into String(format string=w211, initial string=w215, w212, w213, w207) -> (resulting string=w209:string)  [unwired: 1 in, 1 out]
            n111 = Bundle By Name(cluster=T15 {"Value"=0.0, "error"={"status"=FALSE, "code"=0, "source"=""}} ("notification"), "error"=w220, "Value"=w207) -> (w206:T15)
            n112 = local write "Status"(w209) -> ()
            n113 = call "Status Updated.vi"("Status"=w209) -> ()  [unwired: 10 in, 1 out]
            n114 = case shown="True" w208 {
              tunnel: w206 -> [_ w226]
              tunnel: w205 -> [_ w225]
              frame False {
              }
              frame True {
                # "Simulate an operation that requires a wait."
                n115 = flat-sequence {
                  tunnel: w226 -> [w229]
                  tunnel: w225 -> [w228]
                  tunnel: w224 -> [_]
                  frame #0 {
                    n116 = Send Notification(notification=w229, notifier=w228) -> ()  [unwired: 1 in, 2 out]
                  }
                }
                n117 = Wait (ms)(milliseconds to wait=u32 1000) -> (millisecond timer value=w224:u32)
              }
            }
            n118 = Merge Errors(w221, w220) -> (w222:errorcluster)
          }
          frame "Prepare" {
            # "#CodeNeeded\n1. Configure this Message Case for handling the \"Prepare\" message.\n2. Delete or edit this label when done."
            n119 = Variant To Data(error in=w243, type=T8 {"Boolean"=FALSE} ("Prepare Argument"), Variant=w241) -> (error out=w238:errorcluster)  [unwired: 1 out]
            n120 = Open Python Session(python version="3.9" ("Python version"), 3:w238) -> (session out=w236:refnum<k35>, error out=w235:errorcluster)  [unwired: 1 in]
            n121 = Bundle By Name(cluster=w242, "Py Script Path"=path "C:/Projects/579-Intelligent-Systems-Term-Project/06_Source/Python/Scripts/Load-Model_modular.py", "Py Session"=w236) -> (w237:T2)
          }
          frame "Configure" {
            n122 = call "Module Name--constant.vi"() -> ("Module Name"=w255:string)  [unwired: 11 in]
            n123 = call "Create Module Config.vi"("error in"=w246, "DQMH Module Name"=w255) -> ("error out"=w257:errorcluster, "config-ini out"=w256:refnum<class "config-ini.lvclass">)  [unwired: 8 in]
            n124 = control-ref of="This VI"() -> (w248:refnum<vi>)
            n125 = call-dynamic "Read String.vi"("Section"="global" ("global"), "error in"=w257, "Key"="descriptor" ("descriptor"), "config-base in"=w256) -> ("error out"=w252:errorcluster, "Value"=w247:string)  [unwired: 5 in, 1 out]
            n126 = property class="VI"(reference=w248, "Front Panel.Title"=w247) -> ()  [unwired: 1 in, 2 out]
            n127 = call "DQMH System Message - Add to Run-Time Menu.vi"("Module Descriptor"=w247, "Main VI Reference"=w248) -> ("Payload"=w249:variant, "Identifier"=w250:string, "Source"=w251:T17)  [unwired: 7 in]
            n128 = Format Into String(format string="Module %s configured.", w255) -> (resulting string=w253:string)  [unwired: 2 in, 1 out]
            n129 = call "System Message.vi"("Sys. Msg. Source"=w251, "Payload"=w249, "Identifier"=w250) -> ()  [unwired: 8 in, 1 out]
            n130 = call <vilib>:"INFO.vi"("Message"=w253, "error in"=w252) -> ("error out"=w245:errorcluster)  [unwired: 9 in]
            n131 = call "Prepare.vi"("error in"=w245) -> ("error out"=w244:errorcluster)  [unwired: 10 in]
          }
          frame "Request UI Display" {
            n132 = Variant To Data(error in=w273, type=T10 {"Scenario"=enum."Stand-Alone", "Wait Notifier"=refnum, "wait for reply"=FALSE} ("Request UI Display Argument"), Variant=w270) -> (data=w266:T10, error out=w271:errorcluster)
            n133 = Unbundle By Name(w266) -> ("Scenario"=w263:T11, "Wait Notifier"=w261:refnum<notifier>, "wait for reply"=w262:bool)
            n134 = control-ref of="This VI"() -> (w264:refnum<vi>)
            n135 = case shown="\"Managed\"" w263 {
              tunnel: w264 -> [w275 w276]
              tunnel: [w274 w277] -> w265
              frame "Stand-Alone", Default {
                n136 = call "Open VI Panel.vi"("VI"=w275) -> ("error out"=w274:errorcluster)  [unwired: 10 in]
              }
              frame "Managed" {
                n137 = call "DQMH System Message - Ready for Display.vi"("Main VI Reference"=w276) -> ("Payload"=w280:variant, "Identifier"=w279:string, "Source"=w278:T17)  [unwired: 8 in]
                n138 = call "System Message.vi"("Sys. Msg. Source"=w278, "Payload"=w280, "Identifier"=w279) -> ("error out"=w277:errorcluster)  [unwired: 8 in]
              }
            }
            n139 = case shown="True" w262 {
              tunnel: w261 -> [_ w284]
              tunnel: T16 {"Accept"=FALSE, "error"={"status"=FALSE, "code"=0, "source"=""}} ("Request UI Display (Reply Payload)") -> [_ w283]
              tunnel: w265 -> [_ w281]
              frame False {
              }
              frame True {
                n140 = Bundle By Name(cluster=w283, "error"=w281) -> (w282:T16)
                n141 = Send Notification(notification=w282, notifier=w284) -> ()  [unwired: 1 in, 2 out]
              }
            }
            n142 = Merge Errors(w271, w265) -> (w268:errorcluster)
          }
          frame "Update UI" {
            # "#CodeNeeded\n1. Configure this Message Case for handling the \"Update UI\" message.\n2. Delete or edit this label when done."
            # "Sends a request for the module to update the Front Panel controls."
            n143 = Variant To Data(error in=w290, type=T12 {"Update"=FALSE} ("Update UI Argument"), Variant=w288) -> (error out=w289:errorcluster)  [unwired: 1 out]
            n144 = Unbundle By Name(w286) -> ("Status"=→"Status":string)
          }
          frame "---Copy This Frame---" {
            # "Duplicate this frame when creating new messages.  Change this comment in the duplicated frame to describe this message."
            n145 = Merge Errors(w293) -> (w292:errorcluster)
          }
          frame "--- Python ---" {
            # "Duplicate this frame when creating new messages.  Change this comment in the duplicated frame to describe this message."
            n146 = Merge Errors(w296) -> (w295:errorcluster)
          }
          frame "Run MAIN" {
            # "Executes the Main function in Load-Model_modular.py"
            n147 = Unbundle By Name(w307) -> ("Py Session"=w306:refnum<k35>, "Py Script Path"=w305:path)
            n148 = node(w306, w305, "main" ("function name"), w300, "") -> (w299:errorcluster, w301:string)  [unwired: 3 out]
            n149 = Bundle By Name(cluster=w307, "Status"=w301) -> (w302:T2)
            n150 = call "Update UI.vi"("error in"=w299, "Update"=TRUE) -> ("error out"=w298:errorcluster)  [unwired: 9 in]
          }
          frame "---Exit and Error Handling---" {
            # "Separator - The following cases handle errors and exit messages."
          }
          frame "Simulate MHL Error" {
            # "#DQMH_HowTo The 'Simulate MHL Error' button  illustrates how the MHL handles errors. This event is instructional in nature and can be removed."
            # "Simulate an error occurring at the MHL"
            n151 = call "Module Name--constant.vi"() -> ("Module Name"=w311:string)  [unwired: 11 in]
            n152 = Format Into String(format string="Simulated error originating at Message Handling Loop in %s", w311) -> (resulting string=w312:string)  [unwired: 2 in, 1 out]
            n153 = call <vilib>:"Error Cluster From Error Code.vi"("show call chain? (False)"=TRUE, "error message (\"\")"=w312, "error code (0)"=5001) -> ("error out"=w316:errorcluster)  [unwired: 6 in]
            n154 = Merge Errors(w318, w316) -> (w317:errorcluster)
          }
          frame "Error" {
            # "#CodeRecommended - If the module is running in standalone mode (External Launch = FALSE), this code will pop up an error dialog and call the 'Exit' message if an error occurs. Add more fine-grained error management here."
            # "Error - Check the error message data and respond accordingly. This message is sent by the \"Error Handler\" VIs at the end of each loop in this application."
            n155 = property on="Property Node" class="Module Admin"(reference=w323) -> ("Accessors:External Launch"=w322:bool)  [unwired: 1 in, 2 out]
            n156 = Variant To Data(error in=w331, type=errorcluster {"status"=FALSE, "code"=0, "source"=""} ("error constant"), Variant=w325) -> (data=w321:errorcluster, error out=w329:errorcluster)
            n157 = local write "error out"(w321) -> ()
            n158 = call <vilib>:"ERROR.vi"("Message"="DQMH Error Case", "error in"=w321) -> ("error out"=w320:errorcluster)  [unwired: 9 in]
            n159 = call "Error Reported.vi"("Error"=w321) -> ()  [unwired: 10 in, 1 out]
            n160 = case shown="False" w322 {
              tunnel: [w336 _] -> w328
              tunnel: w324 -> [w334 _]
              tunnel: w320 -> [w335 _]
              frame False {
                n161 = disable-structure shown="Default" {
                  disable-tunnel: w335 -> [w337 _]
                  frame condition #0 (active) {
                    # "If the module is running standalone, then pop up an error dialog and call the \"Exit\" message."
                    n162 = call <vilib>:"Simple Error Handler.vi"("error in (no error)"=w337) -> ()  [unwired: 4 in, 5 out]
                  }
                  frame condition #1 {
                    # "To prevent the Simple Error Handler VI from being loaded (e.g. when deploying to a Real-Time target), add the Conditional Disable Symbol \"DQMH_Disable_SEH\" to your project and set it to TRUE."
                  }
                }
                n163 = call-poly <vilib>:"Delacor_lib_QMH_Enqueue Message (poly).vi"("Priority Message? (F)"=TRUE, "Message"="Exit", "Message Queue in"=w334) -> ("error out"=w336:errorcluster)  [unwired: 7 in, 1 out]
              }
              frame True {
                # "If the module was launched externally, calling the Error Reported broadcast VI is the only action performed by the \"Error\" message. The module's caller can then process the error appropriately."
              }
            }
            n164 = Merge Errors(w329, w328) -> (w327:errorcluster)
          }
          frame "Exit" {
            w347 = 91  # 91: not all Exit messages will have an argument
            w349 = TRUE  # Stop the VI
            # "Release the message queue reference"
            # "#CodeNeeded - Add any required cleanup code here."
            # "Exit - Exit the application."
            n165 = Variant To Data(error in=w354, type=T7 {"Origin"="", "Exit via Stop Module Req?"=FALSE, "Wait for Module to stop?"=FALSE} ("Stop Argument"), Variant=w348) -> (data=w345:T7, error out=w342:errorcluster)
            n166 = Unbundle By Name(w339) -> ("Py Session"=w338:refnum<k35>)
            n167 = call <vilib>:"Clear Errors.vi"("error in (no error)"=w342, "specific error code to clear (0: all)"=w347) -> ("error out"=w341:errorcluster)  [unwired: 4 in, 1 out]
            n168 = Close Python Session(session in=w338, error in=w341) -> (11:w340:errorcluster)
            n169 = control-ref of="This VI"() -> (w344:refnum<vi>)
            n170 = call-dynamic "Delacor_lib_QMH_Release Message Queue.vi"("error in"=w340, "Message Queue"=w350) -> ("error out"=w353:errorcluster)  [unwired: 9 in]
            n171 = call "Handle Exit.vi"("Stop Argument"=w345, "Admin in"=w343, "VI reference"=w344) -> ("error out"=w352:errorcluster)  [unwired: 7 in, 1 out]
            n172 = Merge Errors(w353, w352) -> (w351:errorcluster)
            n173 = call "Error Reported.vi"("Error"=w351) -> ()  [unwired: 10 in, 1 out]
          }
          frame Default {
            # "'Default' case only runs if there is a message that isn't defined in any of the other cases.  Output a programming error."
            n174 = call "Module Name--constant.vi"() -> ("Module Name"=w359:string)  [unwired: 11 in]
            n175 = Format Into String(format string="The invalid message string \"%s\" was received in the Message Handling Loop for module \"%s\".", w360, w359) -> (resulting string=w355:string)  [unwired: 2 in, 1 out]
            n176 = call <vilib>:"Error Cluster From Error Code.vi"("show call chain? (False)"=TRUE, "error message (\"\")"=w355, "error code (0)"=1) -> ("error out"=w362:errorcluster)  [unwired: 6 in]
            n177 = Merge Errors(w363, w362) -> (w364:errorcluster)
          }
        }
        n178 = call-dynamic "Delacor_lib_QMH_Error Handler - Message Handling Loop.vi"("error in"=w151, "Message Queue in"=w150) -> ("dup error in"=w152:errorcluster)  [unwired: 8 in, 1 out]
      }
    }
    frame Error {
      # "Synchronize Caller Events.vi will inform Start Module.vi that the module has launched and will let the code calling Start Module.vi register for broadcasts and would permit the caller receive the broadcast that an error occurred at launch time."
      n179 = call-dynamic "Delacor_lib_QMH_Release Message Queue.vi"("error in"=w372, "Message Queue"=w365) -> ("error out"=w371:errorcluster)  [unwired: 9 in]
      n180 = call "Synchronize Caller Events.vi"("Singleton Module Admin in"=w366) -> ("error out"=w373:errorcluster)  [unwired: 9 in, 1 out]
      n181 = call "Module Name--constant.vi"() -> ("Module Name"=w369:string)  [unwired: 11 in]
      n182 = Format Into String(format string="An error occurred during initialization. %s is no longer running.", w369) -> (resulting string=w367:string)  [unwired: 2 in, 1 out]
      n183 = Merge Errors(w371, w373) -> (w374:errorcluster)
      n184 = call "Error Reported.vi"("Additional Information"=w367, "Error"=w374) -> ()  [unwired: 9 in, 1 out]
    }
  }
  n185 = Merge Errors(w18, w21) -> (w17:errorcluster)
  n186 = call "Close Module.vi"("error in"=w17, "Module Admin in"=w12) -> ("error out"=w19:errorcluster, "External Launch"=w5:bool, "Module Admin out"=w6:refnum<class "Delacor_lib_QMH_Module Admin.lvclass">)  [unwired: 7 in]
  n187 = Unregister For Events(event registration refnum=w11, error in=w19) -> (error out=w16:errorcluster)
  n188 = call "Module Name--constant.vi"() -> ("Module Name"=w3:string)  [unwired: 11 in]
  n189 = case "External Launch?" shown="True" w5 {
    tunnel: w16 -> [_ w375]
    frame False {
    }
    frame True {
      n190 = case shown="No Error" w375 {
        frame No Error {
          n191 = invoke on="Invoke Node" class="VI" method="FP.Close"() -> ()  [unwired: 3 in, 3 out]
        }
        frame Error {
          n192 = invoke on="Invoke Node" class="VI" method="FP.Open"("Activate"=TRUE ("Activate?")) -> ()  [unwired: 4 in, 5 out]
        }
      }
    }
  }
  n193 = local write "Module Admin"(w6) -> ()
  n194 = Format Into String(format string="Module %s stopped.", w3) -> (resulting string=w1:string)  [unwired: 2 in, 1 out]
  n195 = call <vilib>:"INFO.vi"("Message"=w1, "error in"=w16) -> ("error out"=→"error out":errorcluster)  [unwired: 9 in]
